vi "connect_to_vsd.vi"(8 "error in (no error)":errorcluster, 10 "vsd":refnum<k24>, 11 "vs_tree_control in":refnum<class "vs_tree_control.lvclass">) -> (0 "error out":errorcluster, 3 "vs_tree_control out":refnum<class "vs_tree_control.lvclass">)   [LabVIEW 2020, in "vs_tree_control.lvclass"]
uses:
  vs_tree_control.lvclass
  vs_tree_control.lvclass/vs_tree_control.ctl
  NationalInstruments.VeriStand.SystemDefinitionAPI
  NationalInstruments.VeriStand.SystemStorageUI
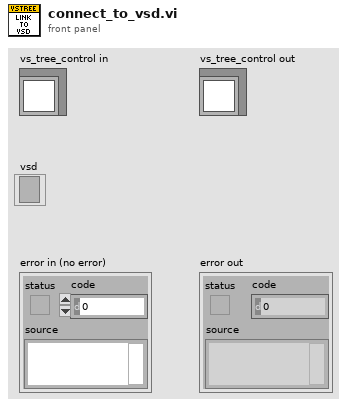
[diagram p1: front panel]
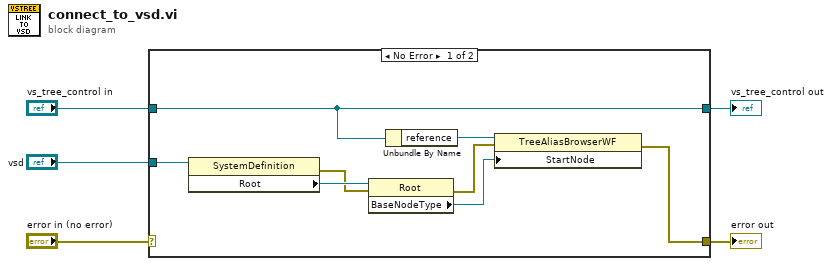
[diagram p0: block diagram]
diagram:
  n1 = case shown="No Error" "error in (no error)" {
    selector: "error in (no error)" -> [_ w15]
    tunnel: [w7 w15] -> w4
    tunnel: [w6 w14] -> w2
    tunnel: "vs_tree_control in" -> [w6 w14]
    tunnel: "vsd" -> [w13 _]
    frame No Error {
      n2 = property class="SystemDefinition"(reference=w13) -> (error out=w11:errorcluster, "Root"=w12:refnum<k24>)  [unwired: 1 in, 1 out]
      n3 = property class="Root"(reference=w12, error in=w11) -> (error out=w8:errorcluster, "BaseNodeType"=w9:refnum<k24>)  [unwired: 1 out]
      n4 = Unbundle By Name(w6) -> ("reference"=w10:refnum<k24>)
      n5 = property class="TreeAliasBrowserWF"(reference=w10, error in=w8, "StartNode"=w9) -> (error out=w7:errorcluster)  [unwired: 1 out]
    }
    frame Error {
    }
  }
  "error out" <- w4
  "vs_tree_control out" <- w2
